vi "ParametersToScript.vi"(8 "error in (no error)":errorcluster, 10 "Params In":string="N/A", 11 "Aerotech_Soloist in":refnum<class "Aerotech_Soloist.lvclass">) -> (0 "error out":errorcluster, 2 "AeroBasic Template Out":string, 3 "Aerotech_Soloist out":refnum<class "Aerotech_Soloist.lvclass">)   [LabVIEW 2013, in "Aerotech_Soloist.lvclass"]
uses:
  Aerotech_Soloist.lvclass
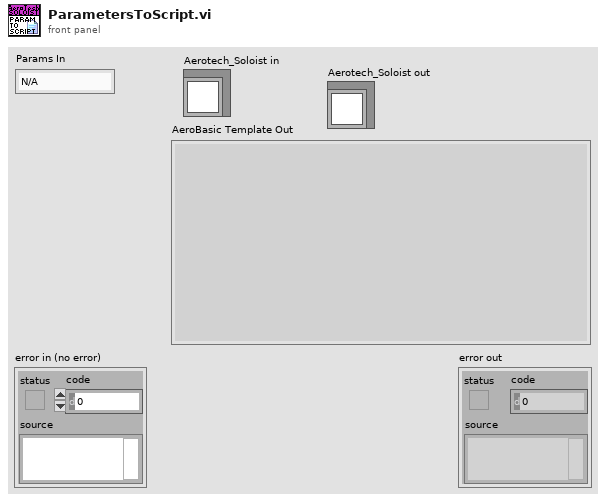
[diagram p1: front panel]
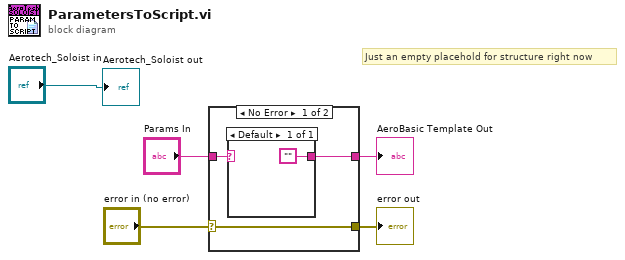
[diagram p0: block diagram]
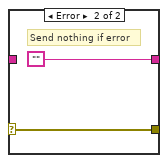
[diagram p2: hidden frame]
diagram:
  # "Just an empty placehold for structure right now"
  n1 = case shown="No Error" "error in (no error)" {
    selector: "error in (no error)" -> [w7 w11]
    tunnel: [w7 w11] -> w4
    tunnel: [w6 ""] -> w3
    tunnel: "Params In" -> [w8 _]
    frame No Error {
      n2 = case shown="Default" w8 {
        tunnel: [""] -> w6
        frame Default {
        }
      }
    }
    frame Error {
      # "Send nothing if error"
    }
  }
  "error out" <- w4
  "AeroBasic Template Out" <- w3
  "Aerotech_Soloist out" <- "Aerotech_Soloist in"
